vi "Config Comparator Mode.vi"(0 "VISA resource name":refnum<visa-resource-name>, 5 "Comparator State (F: OFF)":bool, 7 "Comparator Mode (0: Single)":u16(ring) items=["Single", "Dual"], 11 "error in (no error)":errorcluster) -> (4 "VISA resource name out":refnum<visa-resource-name>, 15 "error out":errorcluster)   [LabVIEW 2016, in "Yokogawa WT200 Series.lvlib"]
doc: "This VI sends the comparator function to the WT200 Series.\n\nNote : It needs /CMP option."
uses:
  Yokogawa WT200 Series.lvlib
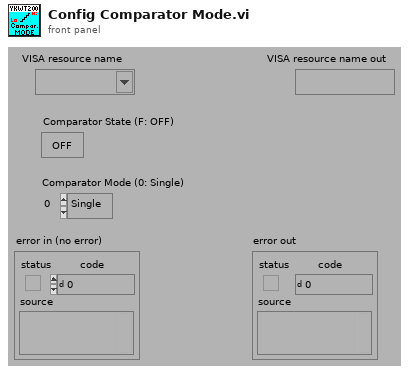
[diagram p1: front panel]
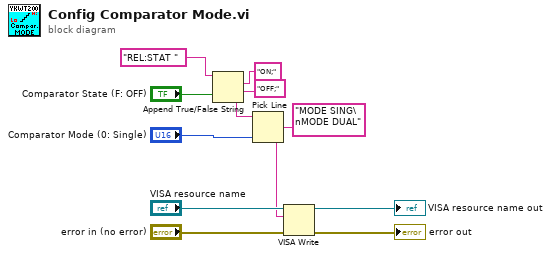
[diagram p0: block diagram]
diagram:
  n1 = Append True/False String(1:"Comparator State (F: OFF)", 2:"OFF;", 3:"ON;", 4:"REL:STAT ") -> (0:w10:string)
  n2 = Pick Line(string ("")=w10, multi-line string="MODE SING\nMODE DUAL", line index="Comparator Mode (0: Single)") -> (output string=w1:string)
  n3 = VISA Write(VISA resource name="VISA resource name", write buffer=w1, error in (no error)="error in (no error)") -> (VISA resource name out=→"VISA resource name out":refnum<visa-resource-name>, error out=→"error out":errorcluster)  [unwired: 1 out]
